vi "Get Category.vi"(8 "error in (no error)":errorcluster, 11 "configuration in":refnum<class "RTResourceUtilitzation configuration.lvclass">) -> (0 "error out":errorcluster, 2 "Category":string, 3 "configuration out":refnum<class "RTResourceUtilitzation configuration.lvclass">)   [LabVIEW 2014, in "RTResourceUtilitzation configuration.lvclass"]
uses:
  RTResourceUtilitzation configuration.lvclass
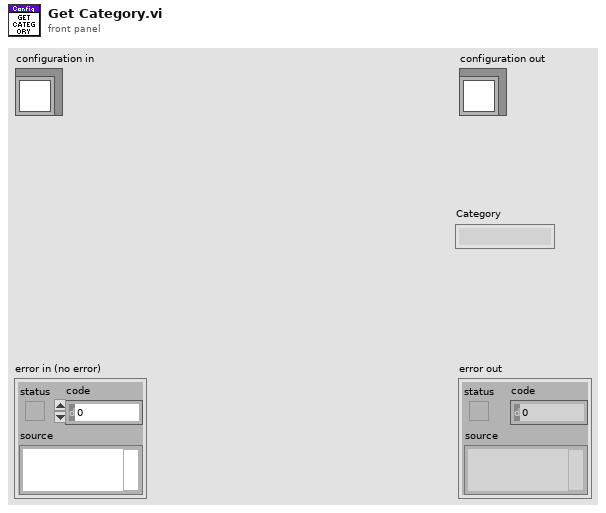
[diagram p1: front panel]
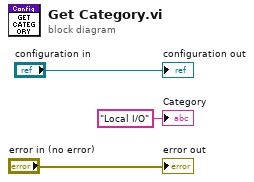
[diagram p0: block diagram]
diagram:
  "error out" <- "error in (no error)"
  "configuration out" <- "configuration in"
  "Category" <- "Local I/O" ("Category")
